vi "Update String Values.vi"(8 "error in (no error)":errorcluster, 10 "Type":u16, 11 "Waveforms Common Methods in":refnum<class "Waveforms Common Methods.lvclass">) -> (0 "error out":errorcluster, 3 "Waveforms Common Methods out":refnum<class "Waveforms Common Methods.lvclass">)   [LabVIEW 2021, in "Rigol DG822 UI.lvlib" / "Waveforms Common Methods.lvclass"]
uses:
  Waveforms Common Methods.lvclass
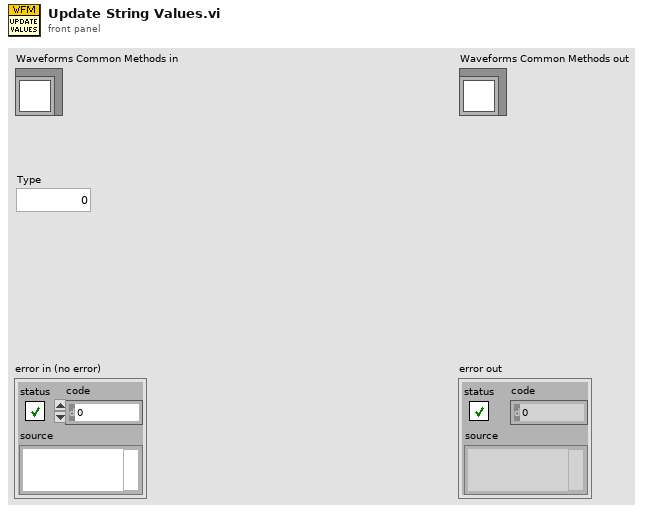
[diagram p1: front panel]
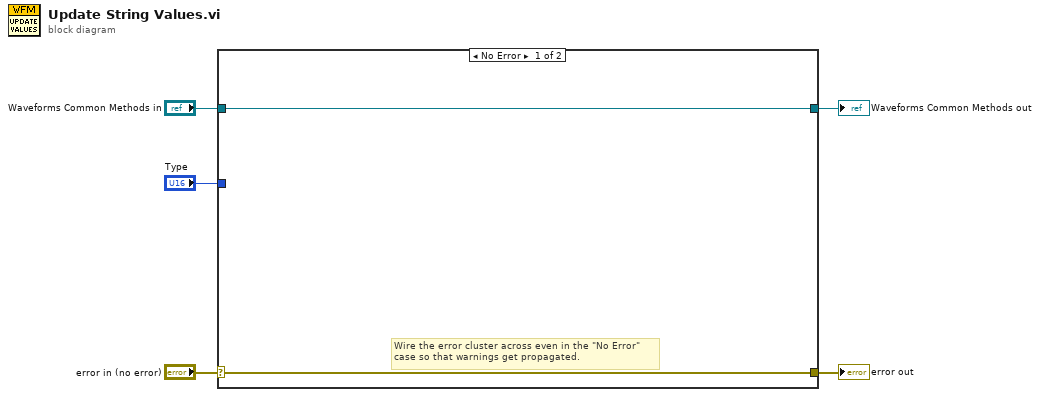
[diagram p0: block diagram]
diagram:
  n1 = case shown="No Error" "error in (no error)" {
    selector: "error in (no error)" -> [w6 w9]
    tunnel: [w6 w9] -> w4
    tunnel: [w7 w8] -> w2
    tunnel: "Waveforms Common Methods in" -> [w7 w8]
    tunnel: "Type" -> [_ _]
    frame No Error {
      # "Wire the error cluster across even in the \"No Error\"\ncase so that warnings get propagated."
    }
    frame Error {
    }
  }
  "error out" <- w4
  "Waveforms Common Methods out" <- w2
